vi "HowToUse.vi"() -> ()   [LabVIEW 2017]
doc: "This VI is just a playground to test Quick Drop's shortcut.\nMake sure, that proper VI is bound to Ctrl+Y shortcut, by pressing Ctrl+space->Configure...->Ctrl-Key Shortcuts."
panel:
  in  "error in (no error) 2":errorcluster
  out "error out 2":errorcluster
  out "error out":errorcluster
  in  "error in (no error)":errorcluster
  # "This QuickDrop shortcut only works on Block Diagram :). \nPress Ctrl+E and see instructions there."
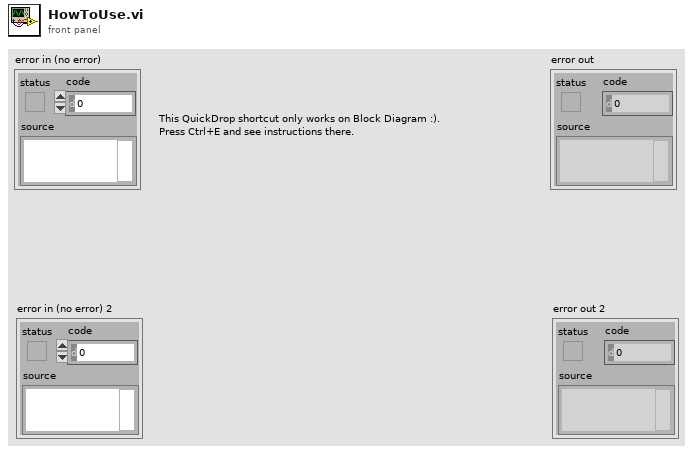
[diagram p1: front panel]
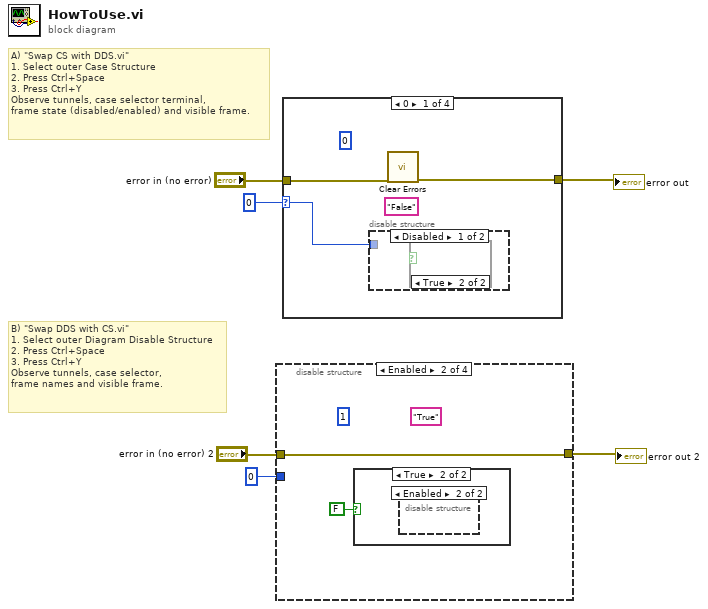
[diagram p0: block diagram]
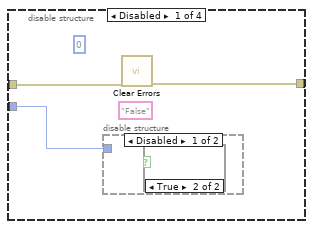
[diagram p2: hidden frame]
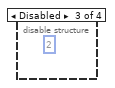
[diagram p7: hidden frame]
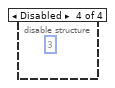
[diagram p8: hidden frame]
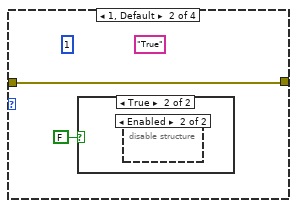
[diagram p11: hidden frame]
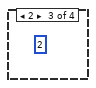
[diagram p14: hidden frame]
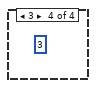
[diagram p15: hidden frame]
diagram:
  # "B) \"Swap DDS with CS.vi\"\n1. Select outer Diagram Disable Structure\n2. Press Ctrl+Space\n3. Press Ctrl+Y\nObserve tunnels, case selector,\nframe names and visible frame."
  # "A) \"Swap CS with DDS.vi\"\n1. Select outer Case Structure\n2. Press Ctrl+Space\n3. Press Ctrl+Y\nObserve tunnels, case selector terminal,\nframe state (disabled/enabled) and visible frame."
  n1 = disable-structure shown="Enabled" {
    disable-tunnel: 0 -> [w9 _ _ _]
    disable-tunnel: [w8 w11 _ _] -> w2
    disable-tunnel: "error in (no error) 2" -> [w7 w11 _ _]
    frame Disabled {
      (unwired) 0
      (unwired) "False"
      n2 = disable-structure shown="Disabled" {
        disable-tunnel: w9 -> [_ _]
        frame Disabled {
          n3 = case shown="True" {
            selector: _ -> [_ _]
            frame False {
            }
            frame True {
            }
          }
        }
        frame Enabled {
        }
      }
      n4 = call <vilib>:"Clear Errors.vi"("error in (no error)"=w7) -> ("error out"=w8:errorcluster)  [unwired: 5 in, 1 out]
    }
    frame Enabled {
      (unwired) 1
      (unwired) "True"
      n5 = case shown="True" FALSE {
        frame False {
        }
        frame True {
          n6 = disable-structure shown="Enabled" {
            frame Disabled {
            }
            frame Enabled {
            }
          }
        }
      }
    }
    frame Disabled {
      (unwired) 2
    }
    frame Disabled {
      (unwired) 3
    }
  }
  "error out 2" <- w2
  n7 = case shown="0" 0 {
    selector: 0 -> [w12 _ _ _]
    tunnel: "error in (no error)" -> [w14 w16 _ _]
    tunnel: [w13 w16 _ _] -> w5
    frame 0 {
      (unwired) 0
      (unwired) "False"
      n8 = disable-structure shown="Disabled" {
        disable-tunnel: w12 -> [_ _]
        frame Disabled {
          n9 = case shown="True" {
            selector: _ -> [_ _]
            frame False {
            }
            frame True {
            }
          }
        }
        frame Enabled {
        }
      }
      n10 = call <vilib>:"Clear Errors.vi"("error in (no error)"=w14) -> ("error out"=w13:errorcluster)  [unwired: 5 in, 1 out]
    }
    frame 1, Default {
      (unwired) 1
      (unwired) "True"
      n11 = case shown="True" FALSE {
        frame False {
        }
        frame True {
          n12 = disable-structure shown="Enabled" {
            frame Disabled {
            }
            frame Enabled {
            }
          }
        }
      }
    }
    frame 2 {
      (unwired) 2
    }
    frame 3 {
      (unwired) 3
    }
  }
  "error out" <- w5
